vi "Free Mem (Mb).vi"() -> (0 "Free Memory (Mb)":dbl format="%.2f")   [LabVIEW 2020]
doc: "Created to just report free memory available. Reports number in Mb (2^20) units.\nScott Hannahs, NHMFL - FSU, December 1995"
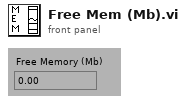
[diagram p1: front panel]
types:
  T1 = cluster{"totalFreeSize":i32, "maxFreeSize":i32, "nFreeblocks":i32, "totAllocSize":i32, "maxAllocSize":i32, "nPointers":i32, "nUnlockedHdls":i32, "nLockedHdls":i32, "reserved1":i32, "reserved2":i32, "reserved3":i32, "reserved4":i32}
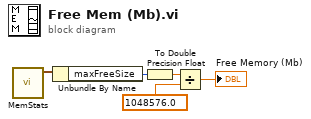
[diagram p0: block diagram]
diagram:
  n1 = call <vilib>:"MemStats.vi"() -> ("AZ memStats"=w2:T1)  [unwired: 5 in, 2 out]
  n2 = Unbundle By Name(w2) -> ("maxFreeSize"=w1:i32)
  n3 = To Double Precision Float(number=w1) -> (double precision float=w3:dbl)
  n4 = Divide(x=w3, y=1048576.0) -> (x/y=→"Free Memory (Mb)":dbl)
